vi "toml_lock_release.vi"(8 "error in (no error)":errorcluster, 11 "lock":refnum<queue>) -> (0 "error out":errorcluster)   [LabVIEW 2017]
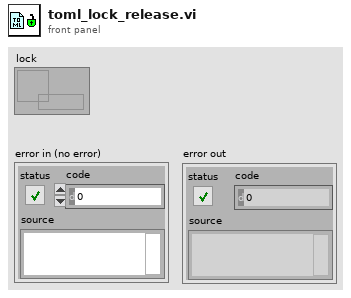
[diagram p1: front panel]
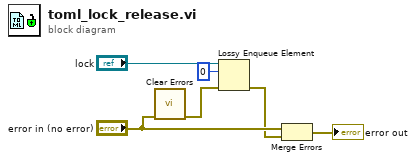
[diagram p0: block diagram]
diagram:
  n1 = call <vilib>:"Clear Errors.vi"("error in (no error)"="error in (no error)") -> ("error out"=w4:errorcluster)  [unwired: 5 in, 1 out]
  n2 = Lossy Enqueue Element(queue="lock", element=u8 0, error in (no error)=w4) -> (error out=w5:errorcluster)  [unwired: 3 out]
  n3 = Merge Errors("error in (no error)", w5) -> (→"error out":errorcluster)
